vi "test color parameters.vi"() -> ()   [LabVIEW 2014, in "AvaSpec.lvlib" / "AvaSpec Acquisition.lvlib"]
uses:
  Acquisition/AvaSpec Acquisition.lvlib
  <vilib>/Utility/file.llb/Read From Spreadsheet File (DBL).vi
  AvaSpec.lvlib
  Acquisition/AvaSpec Color Parameters.ctl
  Acquisition/Sphere Indicator.ctl
panel:
  out "Color Parameters from light matrix":T1 {"Color Values"."v'" format="%#_5g"; "Color Values"."Duv" format="%#_5g"; "Color Values"."u'" format="%#_5g"; "Color Values"."CRI" format="%#_5g"; "Color Values"."CCT" format="%#_5g"; "Color Values"."luminousFlux" format="%#_5g"; "R values" format="%#_4g"; "Tristimulus \nValues"."Z" format="%#_5g"; "Tristimulus \nValues"."Y" format="%#_5g"; "Tristimulus \nValues"."X" format="%#_5g"; "Chromaticity \nCoordinates"."v" format="%#_5g"; "Chromaticity \nCoordinates"."u" format="%#_5g"; "Chromaticity \nCoordinates"."z" format="%#_5g"; "Chromaticity \nCoordinates"."y" format="%#_5g"; "Chromaticity \nCoordinates"."x" format="%#_5g"}
  out "Tristimulus \nValues.X":dbl
  out "Color Parameters self calc":T1 {"Color Values"."v'" format="%#_5g"; "Color Values"."Duv" format="%#_5g"; "Color Values"."u'" format="%#_5g"; "Color Values"."CRI" format="%#_5g"; "Color Values"."CCT" format="%#_5g"; "Color Values"."luminousFlux" format="%#_5g"; "R values" format="%#_4g"; "Tristimulus \nValues"."Z" format="%#_5g"; "Tristimulus \nValues"."Y" format="%#_5g"; "Tristimulus \nValues"."X" format="%#_5g"; "Chromaticity \nCoordinates"."v" format="%#_5g"; "Chromaticity \nCoordinates"."u" format="%#_5g"; "Chromaticity \nCoordinates"."z" format="%#_5g"; "Chromaticity \nCoordinates"."y" format="%#_5g"; "Chromaticity \nCoordinates"."x" format="%#_5g"}
  out "XY Graph":cluster{"X":dbl, "Y":dbl}[](graph)
  # "lum flux and duv off"
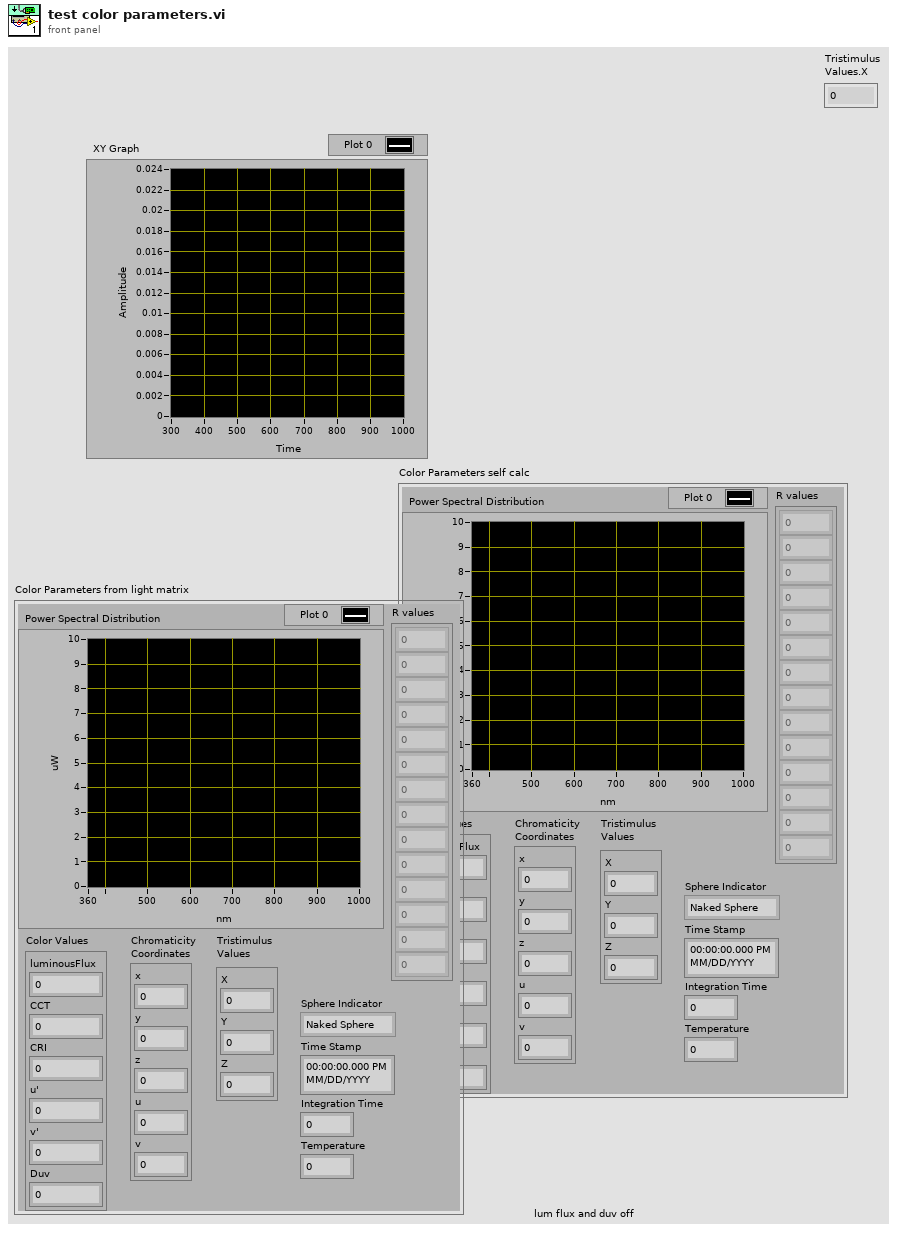
[diagram p1: front panel]
types:
  T1 = typedef "AvaSpec.lvlib/AvaSpec Color Parameters.ctl" = cluster{"Power Spectral Distribution":cluster{"X":dbl, "Y":dbl}[], "Color Values":cluster{"luminousFlux":dbl, "CCT":dbl, "CRI":dbl, "u'":dbl, "v'":dbl, "Duv":dbl}, "R values":dbl[], "Chromaticity \nCoordinates":cluster{"x":dbl, "y":dbl, "z":dbl, "u":dbl, "v":dbl}, "Tristimulus \nValues":cluster{"X":dbl, "Y":dbl, "Z":dbl}, "Time Stamp":timestamp, "Temperature":dbl, "Integration Time":dbl, "Sphere Indicator":T2}
  T2 = typedef "AvaSpec.lvlib/Sphere Indicator.ctl" = enum16{"Naked Sphere", "Insulated Sphere"}
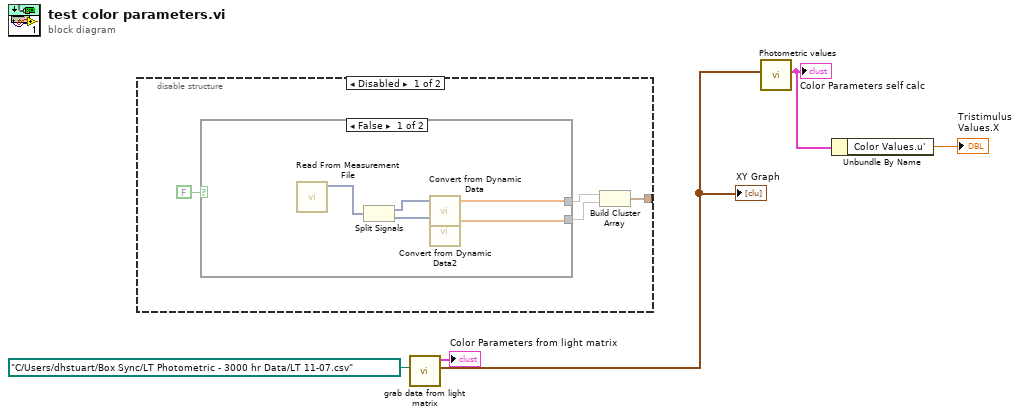
[diagram p0: block diagram]
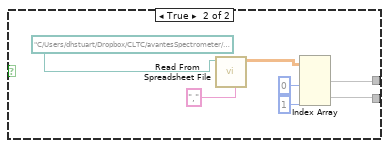
[diagram p2: hidden frame]
diagram:
  n1 = disable-structure shown="Disabled" {
    disable-tunnel: [w6 _] -> _
    frame Disabled {
      n2 = case shown="False" FALSE {
        tunnel: [w11 w16] -> w9
        tunnel: [w10 w15] -> w8
        frame False {
          n3 = call "Read From Measurement File"() -> ("Signals"=w12:dynamicdata)  [unwired: 6 in, 5 out]
          n4 = Split Signals(w12) -> (w13:dynamicdata, w14:dynamicdata)  [unwired: 2 in]
          n5 = call "Convert from Dynamic Data"("Dynamic Data Type"=w13) -> ("Array"=w11:dbl[])  [unwired: 3 in]
          n6 = call "Convert from Dynamic Data2"("Dynamic Data Type"=w14) -> ("Array"=w10:dbl[])  [unwired: 3 in]
        }
        frame True {
          n7 = call-poly <vilib>:"Read From Spreadsheet File.vi"("delimiter (\\t)"="," ("delimiter (\\t)"), "file path (dialog if empty)"=path "C:/Users/dhstuart/Dropbox/CLTC/avantesSpectrometer/irrdata_spectrum_CRI_HiRes.csv") -> ("all rows"=w19:dbl[][])  [unwired: 5 in, 4 out]
          n8 = Index Array(array=w19, index (col) #1=0 ("disabled index (col)"), index (col) #2=1 ("index (col)")) -> (element #1=w16:dbl[], element #2=w15:dbl[])  [unwired: 2 in]
        }
      }
      n9 = Build Cluster Array(w9, w8) -> (w6:cluster{dbl, dbl}[])
    }
    frame Enabled {
    }
  }
  n10 = call "grab data from light matrix.vi"("file path (dialog if empty)"=path "C:/Users/dhstuart/Box Sync/LT Photometric - 3000 hr Data/LT 11-07.csv") -> ("Power Spectral Distribution"=w2:cluster{"X":dbl, "Y":dbl}[], "Color Parameters out"=→"Color Parameters from light matrix":T1)  [unwired: 9 in]
  "XY Graph" <- w2
  n11 = call "Photometric values.vi"("Power Spectral Distribution"=w2) -> ("Color Parameters out"=w5:T1)  [unwired: 9 in, 1 out]
  "Color Parameters self calc" <- w5
  n12 = Unbundle By Name(w5) -> ("Color Values.u'"=→"Tristimulus \nValues.X":dbl)
